vi "ROS2 Close.vi"(6 "error in":errorcluster[](array[cluster]), 9 "DDS in":u64[](array[numeric]), 10 "error in":errorcluster[](array[cluster]), 11 "DDS in":u64[](array[numeric])) -> (0 "error out":errorcluster)   [LabVIEW 2021]
uses:
  <vilib>/RTI DDS Toolkit/Library/LVDDS_library.lvlib
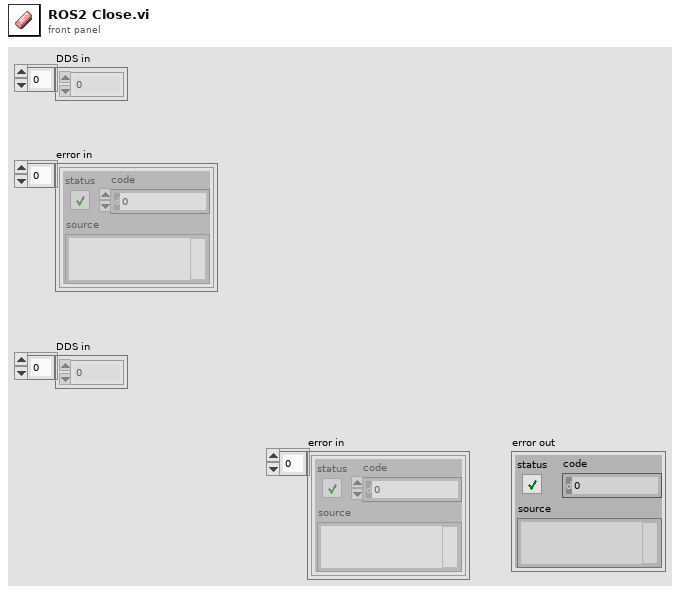
[diagram p1: front panel]
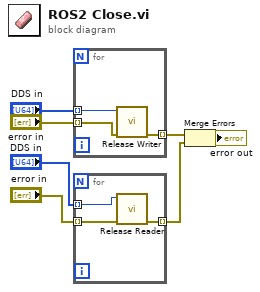
[diagram p0: block diagram]
diagram:
  n1 = for {
    tunnel: [w10] -> w2 mode=indexing
    tunnel: "DDS in" -> [w9] mode=indexing
    tunnel: "error in" -> [w8] mode=indexing
    n2 = call <vilib>:"Release Writer.vi"("error in (no error)"=w8, "DDS Object Ref"=w9) -> ("error out"=w10:errorcluster)  [unwired: 9 in]
  }
  n3 = for {
    tunnel: [w13] -> w3 mode=indexing
    tunnel: "error in" -> [w12] mode=indexing
    tunnel: "DDS in" -> [w11] mode=indexing
    n4 = call <vilib>:"Release Reader.vi"("error in (no error)"=w12, "DDS Object Ref"=w11) -> ("error out"=w13:errorcluster)  [unwired: 9 in]
  }
  n5 = Merge Errors(w2, w3) -> (→"error out":errorcluster)
